vi "VtoC.vi"(1 "Input":dbl[](array[numeric])) -> (0 "Output":dbl[](array[numeric]))   [LabVIEW 2023]
panel:
  out "CJC Temperature (degC)":sgl=25.0 format="%0.2f"
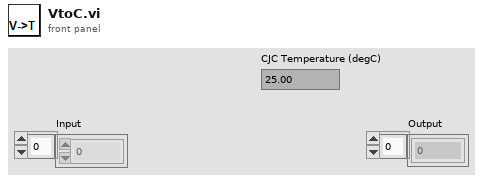
[diagram p1: front panel]
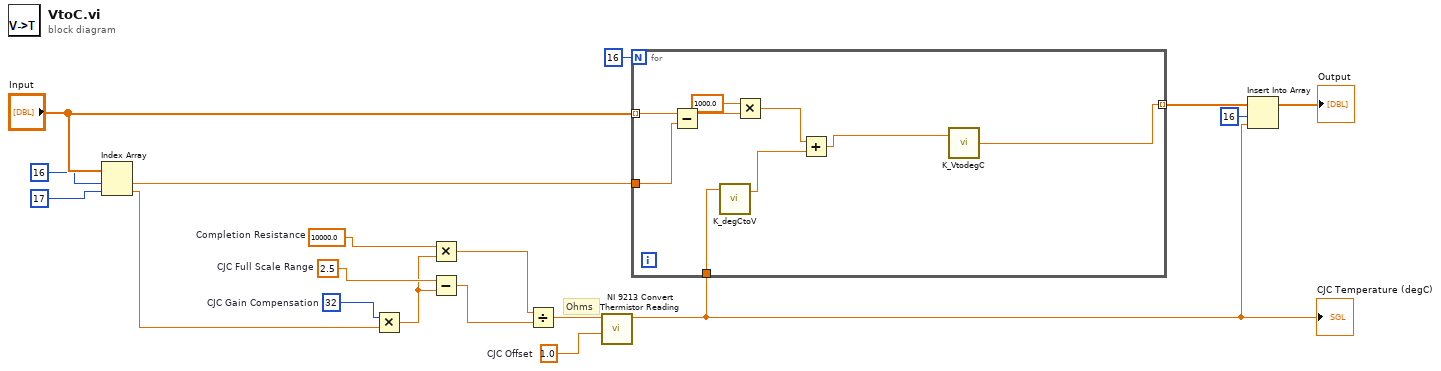
[diagram p0: block diagram]
diagram:
  w11 = 1.0  # CJC Offset
  w15 = sgl 2.5  # CJC Full Scale Range
  w18 = 32  # CJC Gain Compensation
  w16 = sgl 10000.0  # Completion Resistance
  # "Ohms"
  n1 = Index Array(array="Input", index #1=16 ("index"), index #2=17 ("index")) -> (element #1=w4:dbl, element #2=w5:dbl)
  n2 = Multiply(x=w18, y=w5) -> (x*y=w14:dbl)
  n3 = Multiply(x=w16, y=w14) -> (x*y=w12:dbl)
  n4 = Subtract(x=w15, y=w14) -> (x-y=w13:dbl)
  n5 = Divide(x=w12, y=w13) -> (x/y=w17:dbl)
  n6 = call "NI 9213 Convert Thermistor Reading.vi"("CJC Offset"=w11, "Rt"=w17) -> ("CJC Temperature"=w1:sgl)  [unwired: 1 in, 8 out]
  "CJC Temperature (degC)" <- w1
  n7 = for {
    N: 16 -> [_]
    tunnel: [w19] -> w9 mode=indexing
    tunnel: "Input" -> [w27] mode=indexing
    tunnel: w4 -> [w25]
    tunnel: w1 -> [w24]
    n8 = Subtract(x=w27, y=w25) -> (x-y=w26:dbl)
    n9 = call "K_degCtoV.vi"("Temperature (degC)"=w24) -> ("Voltage (mV)"=w21:sgl)  [unwired: 1 in, 1 out]
    n10 = Multiply(x=1000.0, y=w26) -> (x*y=w22:dbl)
    n11 = Add(x=w22, y=w21) -> (x+y=w20:dbl)
    n12 = call "K_VtodegC.vi"("Voltage (mV)"=w20) -> ("Temperature (degC)"=w19:sgl)  [unwired: 1 in]
  }
  n13 = Insert Into Array(array=w9, index=16, new element=w1) -> (→"Output":sgl[])
